vi "SpiralPointsToString.vi"(8 "ZValue":string, 9 "ValveStatus":string, 10 "Typle":string, 11 "Points":cluster{"X":dbl, "Y":dbl}[](array[cluster])) -> (3 "Lines":string[](array[string]))   [LabVIEW 2014]
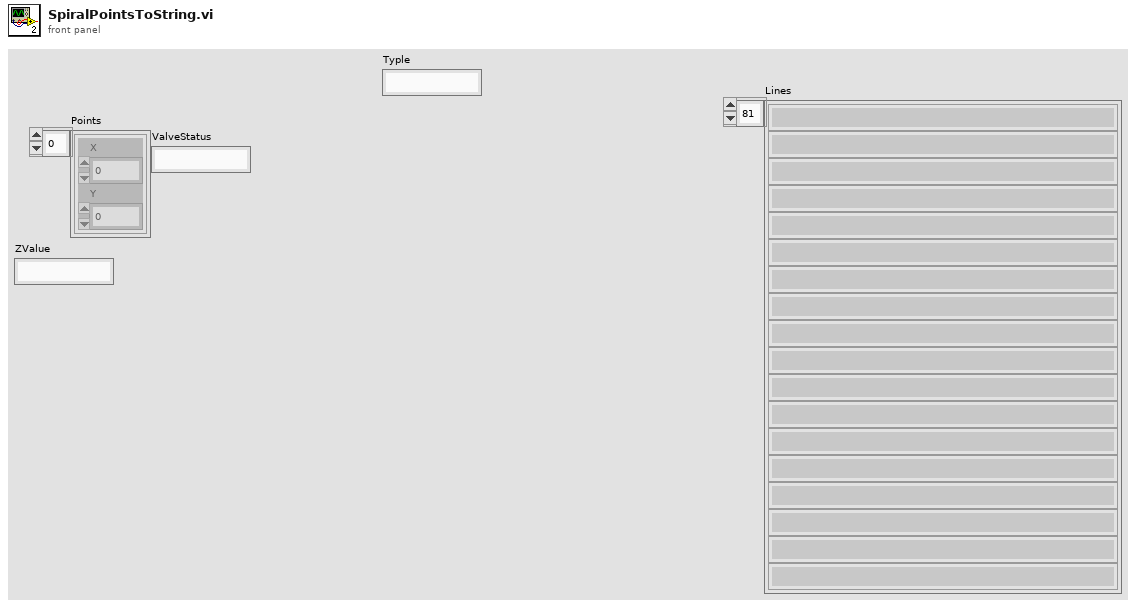
[diagram p1: front panel]
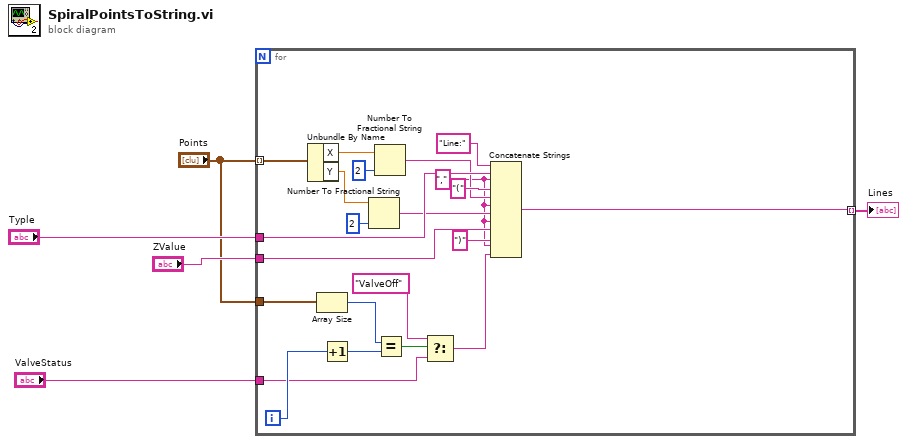
[diagram p0: block diagram]
diagram:
  n1 = for {
    tunnel: "Points" -> [w27] mode=indexing
    tunnel: "Typle" -> [w21]
    tunnel: "ZValue" -> [w17]
    tunnel: "ValveStatus" -> [w9]
    tunnel: "Points" -> [w14]
    tunnel: [w6] -> w1 mode=indexing
    i -> [w12]
    w15 = "," ("字符串")
    n2 = Unbundle By Name(w27) -> ("X"=w26:dbl, "Y"=w23:dbl)
    n3 = Array Size(array=w14) -> (size(s)=w13:i32)
    n4 = Increment(x=w12) -> (x+1=w11:i32)
    n5 = Number To Fractional String(number=w23, precision (6)=i16 2 ("精度(6)")) -> (F-format string=w18:string)  [unwired: 2 in]
    n6 = Number To Fractional String(number=w26, precision (6)=i16 2 ("精度(6)")) -> (F-format string=w19:string)  [unwired: 2 in]
    n7 = Equal?(x=w13, y=w11) -> (x = y?=w10:bool)
    n8 = Select(t="ValveOff", s=w10, f=w9) -> (s? t:f=w7:string)
    n9 = Concatenate Strings("Line:" ("字符串"), w21, w15, "(" ("字符串"), w19, w15, w18, w15, w17, ")" ("字符串"), w15, w7) -> (w6:string)
  }
  "Lines" <- w1
